vi "Bunde ROI info.vi"(0 "ROI Coordinates":i32[](array[numeric]), 1 "ROI Enum":T3, 2 "Z stack Settings":T1, 7 "ZplaneIndex":i32, 9 "Zplanecode":u8) -> (14 "ROI Info":T2={"ROI Enum"=enum."Point", "Coordinates"=[], "Zoom"=1.0, "POI Dwell time"=1.0, "Rel. Resolution"=1.0, "Laser Power"=1.0, "Frame Size"=1.0, "FOV"=1.0, "Z start"=0.0, "Z stop"=0.0, "Z planeIdx(s)"=[], "Z planecodes(s)"=[]} {"FOV" min=1.0 max=10.0 step=1.0; "Frame Size" min=1.0 max=10.0 step=1.0; "Laser Power" min=1.0 max=10.0 step=0.10000000149011612; "Rel. Resolution" min=1.0 max=10.0 step=1.0; "POI Dwell time" min=1.0 max=10.0 step=0.10000000149011612; "Zoom" min=1.0 max=10.0 step=0.10000000149011612})   [LabVIEW 2020]
uses:
  Typedefs/ROI ID Enum.ctl
  Typedefs/ROI spec.ctl
  ROI Entry screen/Typedefs/ROI Z-stack settings info.ctl
panel:
  in  "FOV":dbl
  in  "Frame Size":dbl
  in  "Laser Power":dbl
  in  "Rel. Resolution":dbl
  in  "POI Dwell time":dbl
  in  "Zoom":dbl
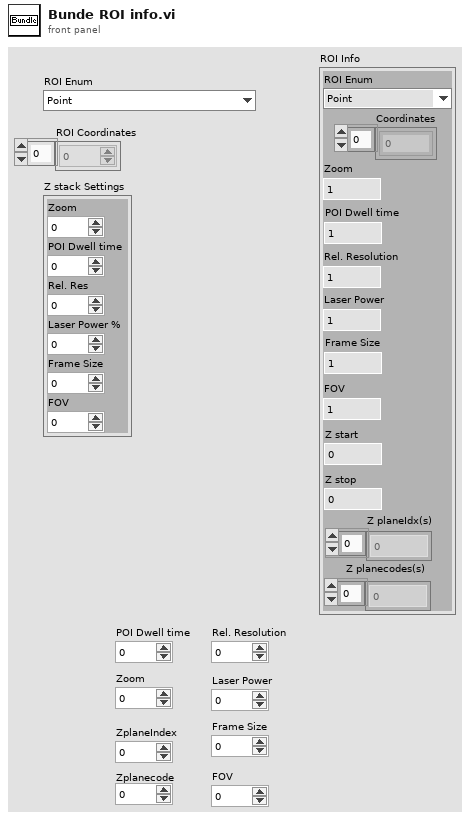
[diagram p1: front panel]
types:
  T1 = typedef "ROI Z-stack settings info.ctl" = cluster{"Zoom":dbl, "POI Dwell time":dbl, "Rel. Res":dbl, "Laser Power %":dbl, "Frame Size":dbl, "FOV":dbl}
  T2 = typedef "ROI spec.ctl" = cluster{"ROI Enum":T3, "Coordinates":i32[], "Zoom":dbl, "POI Dwell time":dbl, "Rel. Resolution":dbl, "Laser Power":dbl, "Frame Size":dbl, "FOV":dbl, "Z start":dbl, "Z stop":dbl, "Z planeIdx(s)":i32[], "Z planecodes(s)":u8[]}
  T3 = typedef "ROI ID Enum.ctl" = enum16{"Point", "MiniScan", "Comp. MiniScan", "Rectangle", "Comp. volume", "Arb. plane point", "None"}
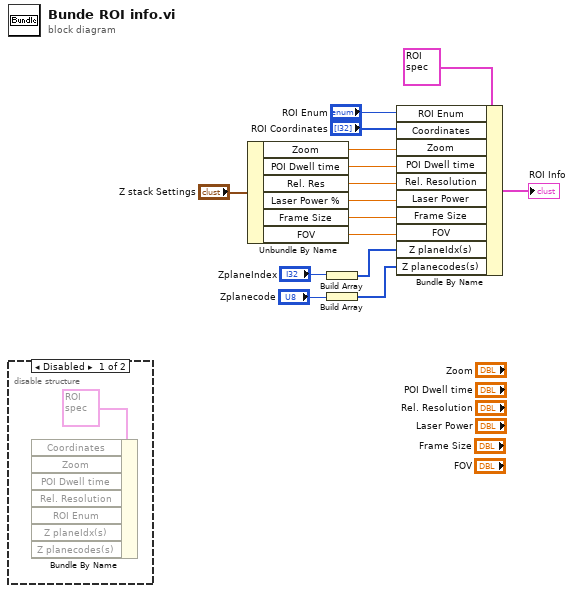
[diagram p0: block diagram]
diagram:
  n1 = disable-structure shown="Disabled" {
    frame Disabled {
      n2 = Bundle By Name(cluster=T2 {"ROI Enum"=enum."Point", "Coordinates"=[], "Zoom"=1.0, "POI Dwell time"=1.0, "Rel. Resolution"=1.0, "Laser Power"=1.0, "Frame Size"=1.0, "FOV"=1.0, "Z start"=0.0, "Z stop"=0.0, "Z planeIdx(s)"=[], "Z planecodes(s)"=[]} ("input cluster")) -> ("Z planecodes(s)"=w16:u8[])  [unwired: 6 in, 1 out]
    }
    frame Enabled {
    }
  }
  n3 = Unbundle By Name("Z stack Settings") -> ("Zoom"=w6:dbl, "POI Dwell time"=w5:dbl, "Rel. Res"=w4:dbl, "Laser Power %"=w3:dbl, "Frame Size"=w2:dbl, "FOV"=w1:dbl)
  n4 = Build Array("ZplaneIndex") -> (w9:i32[])
  n5 = Build Array("Zplanecode") -> (w8:u8[])
  n6 = Bundle By Name(cluster=T2 {"ROI Enum"=enum."Point", "Coordinates"=[], "Zoom"=1.0, "POI Dwell time"=1.0, "Rel. Resolution"=1.0, "Laser Power"=1.0, "Frame Size"=1.0, "FOV"=1.0, "Z start"=0.0, "Z stop"=0.0, "Z planeIdx(s)"=[], "Z planecodes(s)"=[]} ("input cluster"), "ROI Enum"="ROI Enum", "Coordinates"="ROI Coordinates", "Zoom"=w6, "POI Dwell time"=w5, "Rel. Resolution"=w4, "Laser Power"=w3, "Frame Size"=w2, "FOV"=w1, "Z planeIdx(s)"=w9, "Z planecodes(s)"=w8) -> (→"ROI Info":T2)
